vi "Global_SM Out Data.vi"() -> ()   [LabVIEW 2017, in "WCDrive2018.lvlib"]
uses:
  WCDrive2018.lvlib
  Cluster_SM Status.ctl
  Enum_SM Cmd Select.ctl
  Cluster_SM to HW Data.ctl
  Enum_HW Cmd Select.ctl
panel:
  in  "Drive_SM_HWCmd":T1
  in  "Drive_SM_Status":T3
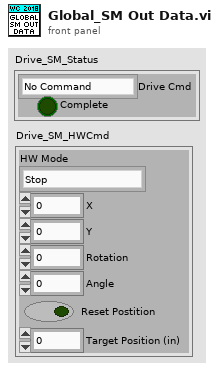
[diagram p1: front panel]
types:
  T1 = typedef "WCDrive2018.lvlib/Cluster_SM to HW Data.ctl" = cluster{"HW Mode":T2, "X":dbl, "Y":dbl, "Rotation":dbl, "Angle":dbl, "Reset Postition":bool, "Target Position (in)":dbl}
  T2 = typedef "WCDrive2018.lvlib/Enum_HW Cmd Select.ctl" = enum16{"Stop", "Vbus", "Positon Lateral", "Postition  FrontBack"}
  T3 = typedef "WCDrive2018.lvlib/Cluster_SM Status.ctl" = cluster{"Drive Cmd":T4, "Complete":bool}
  T4 = typedef "WCDrive2018.lvlib/Enum_SM Cmd Select.ctl" = enum16{"No Command", "Halt", "Manual Keep Rotation", "Manual", "Track Front", "Track Rotation"}
diagram:
